vi "Cam Response Vi.vi"(7 "state":T1, 8 "error in":errorcluster, 10 "Module ID":i32=-1, 11 "recived ID":refnum<k5>) -> (0 "error out":errorcluster, 3 "recived ID 2":refnum<k5>)   [LabVIEW 2024, in "cameraV1.lvlib"]
uses:
  cameraV1.lvlib
  Controls/state.ctl
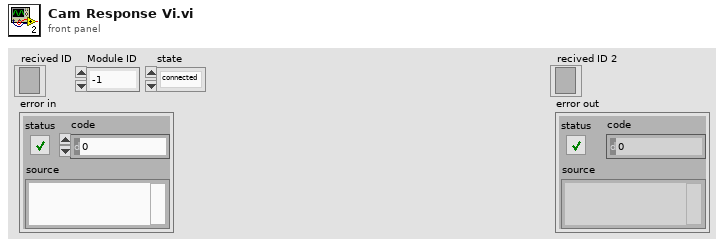
[diagram p1: front panel]
types:
  T1 = typedef "cameraV1.lvlib/state.ctl" = enum16{"connected", "not connected", "Online", "Offline"}
  T2 = enum16{"Standard", "Buffered", "CRLF", "Immediate"}
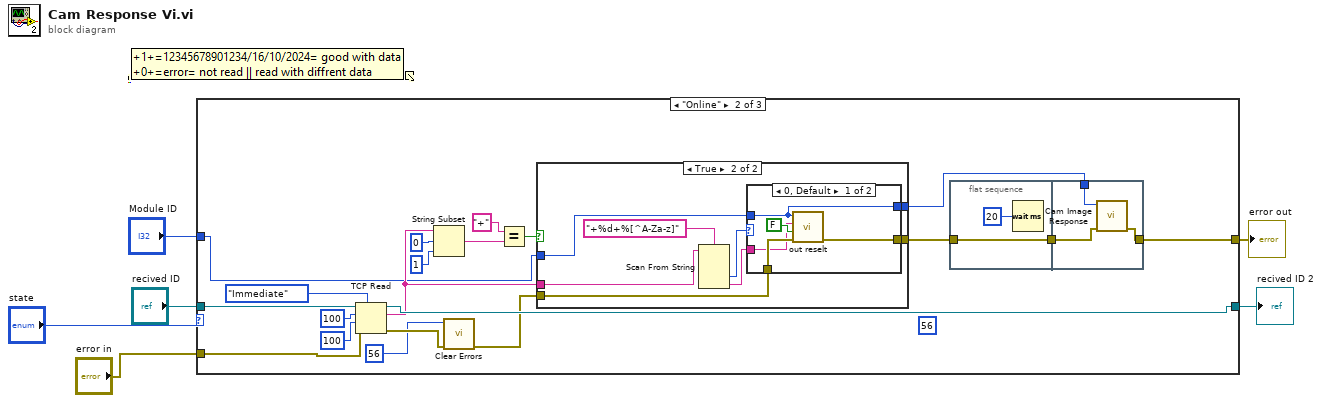
[diagram p0: block diagram]
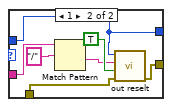
[diagram p4: hidden frame]
diagram:
  n1 = case shown="\"Online\"" "state" {
    tunnel: "recived ID" -> [w8 w26 w57]
    tunnel: [w8 w25 w57] -> w5
    tunnel: "Module ID" -> [_ w17 _]
    tunnel: [w7 w10 w56] -> w2
    tunnel: "error in" -> [w7 w13 w56]
    frame "connected", Default {
    }
    frame "Online" {
      (unwired) 56 ("specific error code to clear (0: all)")
      n2 = TCP Read(connection ID=w26, bytes to read=100, error in (no error)=w13, 7:T2."Immediate" ("mode (standard)"), 9:100 ("timeout ms (25000)")) -> (connection ID out=w25:refnum<k5>, data out=w19:string, error out=w16:errorcluster)
      n3 = String Subset(string=w19, offset (0)=0, length (rest)=1 ("length (rest)")) -> (substring=w22:string)
      n4 = call <vilib>:"Clear Errors.vi"("error in (no error)"=w16, "specific error code to clear (0: all)"=56) -> ("error out"=w14:errorcluster)  [unwired: 4 in, 1 out]
      n5 = Equal?(x="+", y=w22) -> (x = y?=w20:bool)
      n6 = case shown="True" w20 {
        tunnel: w19 -> [_ w37]
        tunnel: w17 -> [w29 w35]
        tunnel: w14 -> [w30 w34]
        tunnel: [w30 w33] -> w12
        tunnel: [w29 w31] -> w9
        frame False {
        }
        frame True {
          n7 = Scan From String(format string="+%d+%[^A-Za-z]", input string=w37) -> (output 1=w36:i32, output 2=w32:string)  [unwired: 4 in, 3 out]
          n8 = case shown="0, Default" w36 {
            tunnel: w35 -> [w39 w44]
            tunnel: w34 -> [w42 w46]
            tunnel: [w41 w45] -> w33
            tunnel: w32 -> [w40 w50]
            tunnel: [w39 w44] -> w31
            frame 0, Default {
              n9 = call "out reselt.vi"("error in"=w42, "status"=FALSE, "serial"=w40, "Module ID"=w39) -> ("error out"=w41:errorcluster)  [unwired: 7 in]
            }
            frame 1 {
              n10 = Match Pattern(string=w50, regular expression="/") -> (after substring=w47:string)  [unwired: 1 in, 3 out]
              n11 = call "out reselt.vi"("error in"=w46, "status"=TRUE, "serial"=w47, "Module ID"=w44) -> ("error out"=w45:errorcluster)  [unwired: 7 in]
            }
          }
        }
      }
      n12 = flat-sequence {
        tunnel: w12 -> [w51]
        tunnel: [w51] -> w11
        tunnel: w11 -> [w55]
        tunnel: [w54] -> w10
        tunnel: w9 -> [w53]
        frame #0 {
          n13 = Wait (ms)(milliseconds to wait=u32 20) -> ()  [unwired: 1 out]
        }
        frame #1 {
          n14 = call "Cam Image Response.vi"("error in"=w55, "Module ID"=w53) -> ("error out"=w54:errorcluster)  [unwired: 9 in]
        }
      }
    }
    frame "Offline" {
    }
  }
  "recived ID 2" <- w5
  "error out" <- w2
